vi "GetAAStatus.vi"(5 "error in":T1) -> (14 "State out":i32, 19 "error out":T1)   [LabVIEW 2016]
doc: "Returns the current status of auto approach (1 = on; 0 = off)."
uses:
  Controls/Error_Out.ctl
  Files_ASC500/DLL/ASC500_RemoteControlV27.dll
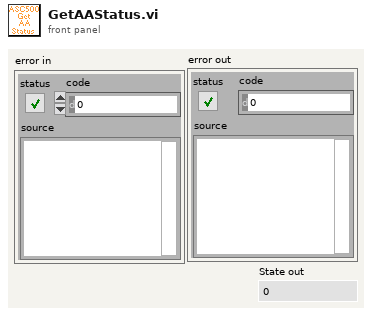
[diagram p1: front panel]
types:
  T1 = typedef "Error_Out.ctl" = errorcluster
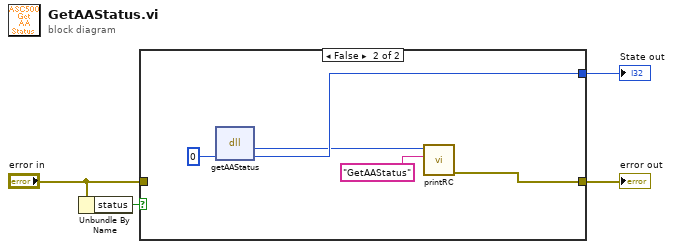
[diagram p0: block diagram]
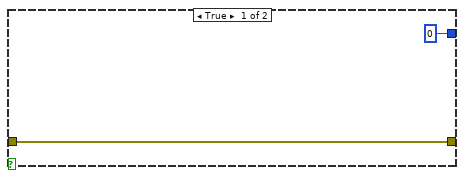
[diagram p2: hidden frame]
diagram:
  n1 = Unbundle By Name("error in") -> ("status"=w4:bool)
  n2 = case shown="False" w4 {
    tunnel: [0 ("Status") w10] -> w3
    tunnel: "error in" -> [w5 _]
    tunnel: [w5 w9] -> w1
    frame True {
    }
    frame False {
      n3 = dll-call lib="G:/SCMOperations/Share/ELE/Produkt Information/ASC500/04 Remote Control/02 development versions/2018Nov06/Files_ASC500/DLL/ASC500_RemoteControlV27.dll" fn="getAAStatus"("Status"=0) -> ("return type"=w8:i32, "Status"=w10:i32)  [unwired: 3 in, 2 out]
      n4 = call "printRC.vi"("additional information"="GetAAStatus", "RC"=w8) -> ("error out"=w9:T1)  [unwired: 9 in]
    }
  }
  "error out" <- w1
  "State out" <- w3
